vi "set_process_priority.vi"(8 "error in (no error)":errorcluster, 10 "PriorityClass":i32(ring)=32 items=["Normal"=32, "Idle"=64, "High"=128, "RealTime"=256, "BelowNormal"=16384, "AboveNormal"=32768]) -> (0 "error out":errorcluster)   [LabVIEW 2010]
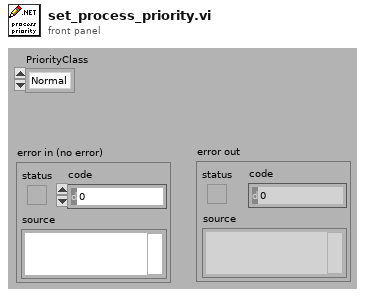
[diagram p1: front panel]
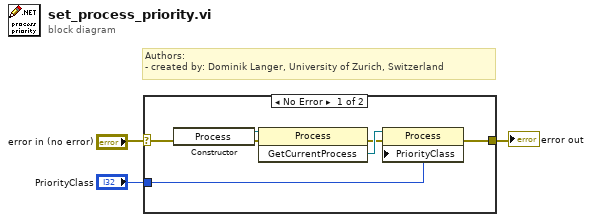
[diagram p0: block diagram]
diagram:
  # "Authors: \n- created by: Dominik Langer, University of Zurich, Switzerland"
  n1 = case shown="No Error" "error in (no error)" {
    selector: "error in (no error)" -> [w6 w11]
    tunnel: [w5 w11] -> w2
    tunnel: "PriorityClass" -> [w4 _]
    frame No Error {
      n2 = constructor class="Process"(error in=w6) -> (reference out=w10:refnum<k24>, error out=w8:errorcluster)  [unwired: 2 in, 1 out]
      n3 = invoke class="Process" method="GetCurrentProcess"(reference=w10, error in=w8) -> (error out=w7:errorcluster, "GetCurrentProcess"=w9:refnum<k24>)  [unwired: 1 in, 1 out]
      n4 = property class="Process"(reference=w9, error in=w7, "PriorityClass"=w4) -> (error out=w5:errorcluster)  [unwired: 1 out]
    }
    frame Error {
    }
  }
  "error out" <- w2
